vi "Stop.vi"(10 "Code":i32, 11 "Test 1 in":refnum<class "Test 1.lvclass">) -> (3 "Test 1 out":refnum<class "Test 1.lvclass">)   [LabVIEW 2020, in "Scratchpad.lvlib" / "Test 1.lvlib" / "Test 1.lvclass"]
uses:
  Test 1.lvclass
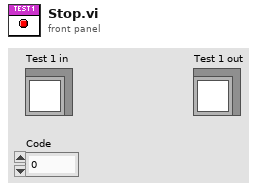
[diagram p1: front panel]
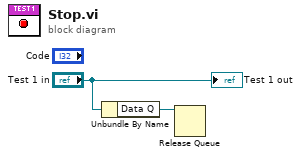
[diagram p0: block diagram]
diagram:
  n1 = Unbundle By Name("Test 1 in") -> ("Data Q"=w1:refnum<queue>)
  n2 = Release Queue(queue=w1) -> ()  [unwired: 2 in, 3 out]
  "Test 1 out" <- "Test 1 in"
